vi "Load Config.vi"(8 "error in (no error)":errorcluster, 11 "RTDChannel in":refnum<class "RTDChannel.lvclass">) -> (0 "error out":errorcluster, 3 "RTDChannel out":refnum<class "RTDChannel.lvclass">)   [LabVIEW 2020, in "VolatusDAQConfig.lvlib" / "RTDChannel.lvclass"]
uses:
  RTDChannel.lvclass
  RTDChannel.lvclass/RTDChannel.ctl
  VolatusConfig/VolatusConfigElement/VolatusConfigElement.lvclass
  lv-cdm/CDM-Config/Config Element/Config Element.lvclass
  RTD Excitation.ctl
  VolatusDAQConfig.lvlib
  C:/dev/lv20CE/relink/lv-volatus/VolatusDAQConfig/DAQmxChannel/DAQmxChannel.lvclass
  C:/dev/lv20CE/relink/lv-volatus/VolatusConfig/Channel/Channel.lvclass
  C:/dev/lv20CE/relink/lv-volatus/VolatusConfig/VolatusConfigElement/VolatusConfigElement.lvclass
  C:/dev/lv20CE/relink/lv-volatus/VolatusDAQConfig/RTDChannel/RTDChannel.lvclass
  RTD Wiring.ctl
  Temperature Units.ctl
  RTD Type.ctl
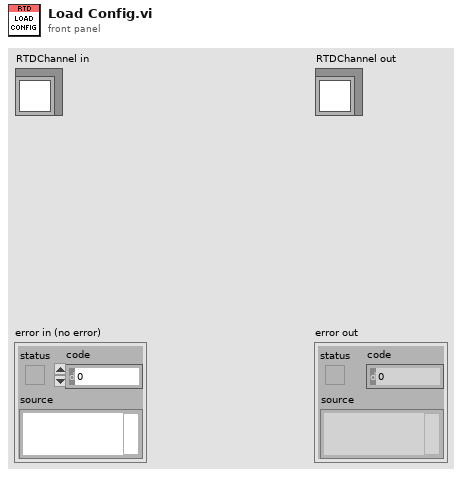
[diagram p1: front panel]
types:
  T1 = typedef "VolatusDAQConfig.lvlib/RTD Type.ctl" = enum16{"Pt3750", "Pt3851", "Pt3911", "Pt3916", "Pt3920", "Pt3928", "Custom"}
  T2 = typedef "VolatusDAQConfig.lvlib/Temperature Units.ctl" = enum16{"C", "F", "K", "R"}
  T3 = typedef "VolatusDAQConfig.lvlib/RTD Wiring.ctl" = enum16{"2-Wire", "3-Wire", "4-Wire"}
  T4 = typedef "VolatusDAQConfig.lvlib/RTD Excitation.ctl" = enum16{"Internal", "External", "None"}
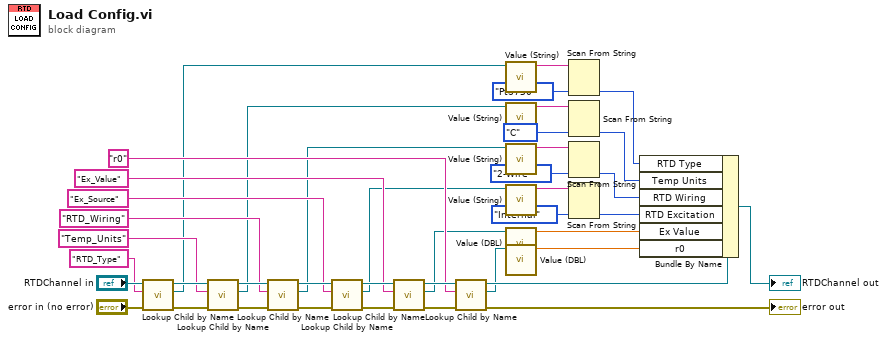
[diagram p0: block diagram]
diagram:
  n1 = call "Lookup Child by Name.vi"("error in (no error)"="error in (no error)", "Child Name"="RTD_Type", "VolatusConfigElement in"="RTDChannel in") -> ("error out"=w40:errorcluster, "Child"=w16:refnum<class "Config Element.lvclass">, "VolatusConfigElement out"=w36:refnum<class "RTDChannel.lvclass">)  [unwired: 5 in, 1 out]
  n2 = call "Lookup Child by Name.vi"("error in (no error)"=w40, "Child Name"="Temp_Units", "VolatusConfigElement in"=w36) -> ("error out"=w37:errorcluster, "Child"=w17:refnum<class "Config Element.lvclass">, "VolatusConfigElement out"=w33:refnum<class "RTDChannel.lvclass">)  [unwired: 5 in, 1 out]
  n3 = call "Lookup Child by Name.vi"("error in (no error)"=w37, "Child Name"="RTD_Wiring", "VolatusConfigElement in"=w33) -> ("error out"=w34:errorcluster, "Child"=w18:refnum<class "Config Element.lvclass">, "VolatusConfigElement out"=w30:refnum<class "RTDChannel.lvclass">)  [unwired: 5 in, 1 out]
  n4 = call "Lookup Child by Name.vi"("error in (no error)"=w34, "Child Name"="Ex_Source", "VolatusConfigElement in"=w30) -> ("error out"=w31:errorcluster, "Child"=w19:refnum<class "Config Element.lvclass">, "VolatusConfigElement out"=w27:refnum<class "RTDChannel.lvclass">)  [unwired: 5 in, 1 out]
  n5 = call "Lookup Child by Name.vi"("error in (no error)"=w31, "Child Name"="Ex_Value", "VolatusConfigElement in"=w27) -> ("error out"=w28:errorcluster, "Child"=w20:refnum<class "Config Element.lvclass">, "VolatusConfigElement out"=w24:refnum<class "RTDChannel.lvclass">)  [unwired: 5 in, 1 out]
  n6 = call "Lookup Child by Name.vi"("error in (no error)"=w28, "Child Name"="r0", "VolatusConfigElement in"=w24) -> ("error out"=→"error out":errorcluster, "Child"=w21:refnum<class "Config Element.lvclass">, "VolatusConfigElement out"=w23:refnum<class "RTDChannel.lvclass">)  [unwired: 5 in, 1 out]
  n7 = call "Value (String).vi"("Config Element in"=w16) -> ("String Value"=w15:string)  [unwired: 9 in, 1 out]
  n8 = call "Value (String).vi"("Config Element in"=w17) -> ("String Value"=w14:string)  [unwired: 9 in, 1 out]
  n9 = call "Value (String).vi"("Config Element in"=w18) -> ("String Value"=w13:string)  [unwired: 9 in, 1 out]
  n10 = call "Value (String).vi"("Config Element in"=w19) -> ("String Value"=w12:string)  [unwired: 9 in, 1 out]
  n11 = call "Value (DBL).vi"("Config Element in"=w20) -> ("DBL Value"=w9:dbl)  [unwired: 9 in, 1 out]
  n12 = call "Value (DBL).vi"("Config Element in"=w21) -> ("DBL Value"=w10:dbl)  [unwired: 9 in, 1 out]
  n13 = Scan From String(input string=w15, default 1=RTD_Type."Pt3750" ("RTD Type")) -> (output 1=w5:T1)  [unwired: 3 in, 3 out]
  n14 = Scan From String(input string=w14, default 1=Temperature_Units."C" ("Temp Units")) -> (output 1=w6:T2)  [unwired: 3 in, 3 out]
  n15 = Scan From String(input string=w13, default 1=RTD_Wiring."2-Wire" ("RTD Wiring")) -> (output 1=w7:T3)  [unwired: 3 in, 3 out]
  n16 = Scan From String(input string=w12, default 1=RTD_Excitation."Internal" ("RTD Excitation")) -> (output 1=w8:T4)  [unwired: 3 in, 3 out]
  n17 = Bundle By Name(cluster=w23, "RTD Type"=w5, "Temp Units"=w6, "RTD Wiring"=w7, "RTD Excitation"=w8, "Ex Value"=w9, "r0"=w10) -> (→"RTDChannel out":refnum<class "RTDChannel.lvclass">)
